vi "get display data.vi"(0 "display queues":T4, 1 "prune?":bool=TRUE, 5 "time range":dbl=-1.0, 9 "t0":dbl, 11 "error in (no error)":errorcluster, 12 "recent crossing":dbl) -> (4 "voltage graph":cluster{dbl[], dbl[]}, 6 "coil graph":cluster{dbl[], dbl[]}, 8 "pulse statistics":T1, 10 "extracted magnetism":T2[](array[typedef]), 15 "error out":errorcluster)   [LabVIEW 2017]
uses:
  typedefs/queue cluster.ctl
  typedefs/reading queue.ctl
  typedefs/reading.ctl
  typedefs/readingType.ctl
  typedefs/reading1.ctl
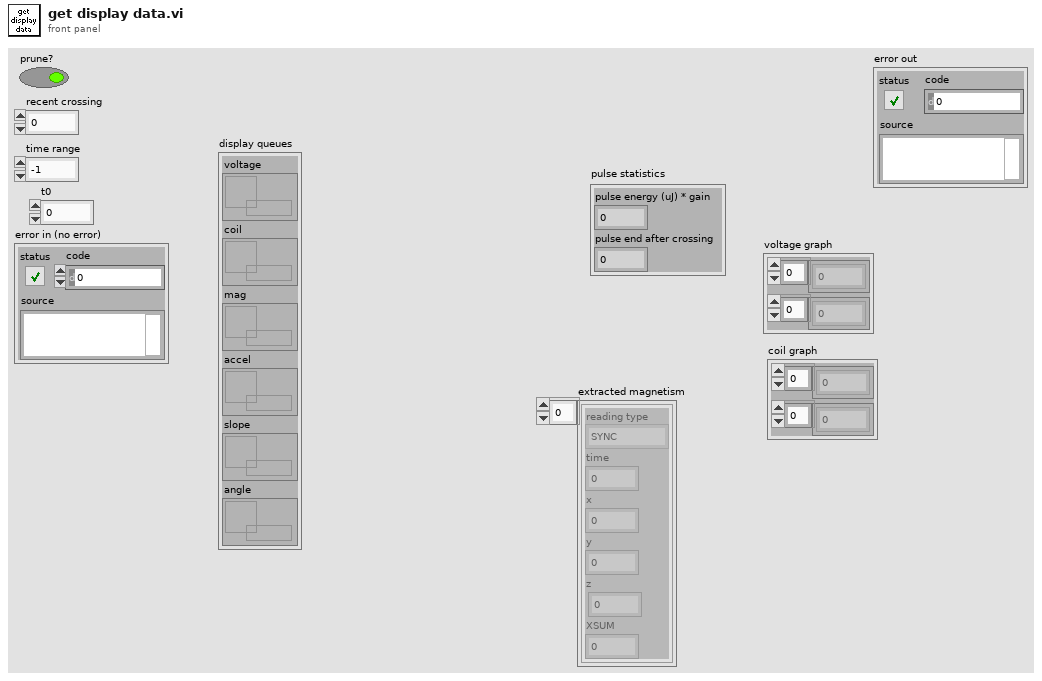
[diagram p1: front panel]
types:
  T1 = cluster{"pulse energy (uJ) * gain":sgl, "pulse end after crossing":dbl}
  T2 = typedef "reading.ctl" = cluster{"reading type":T3, "time":fxp<+,48,48>, "x":sgl, "y":sgl, "z":sgl, "XSUM":u8}
  T3 = typedef "readingType.ctl" = enum8{"SYNC", "DETVAL", "COILI", "MAGVEC", "ACCVEC"}
  T4 = typedef "queue cluster.ctl" = cluster{"voltage":T5, "coil":T5, "mag":T5, "accel":T5, "slope":refnum<queue>, "angle":refnum<queue>}
  T5 = typedef "reading queue.ctl" = refnum<queue>
  T6 = cluster{"tx":cluster{dbl[], sgl[]}, "ty":cluster{dbl[], sgl[]}, "tz":cluster{dbl[], sgl[]}, "xy":cluster{sgl[], sgl[]}}
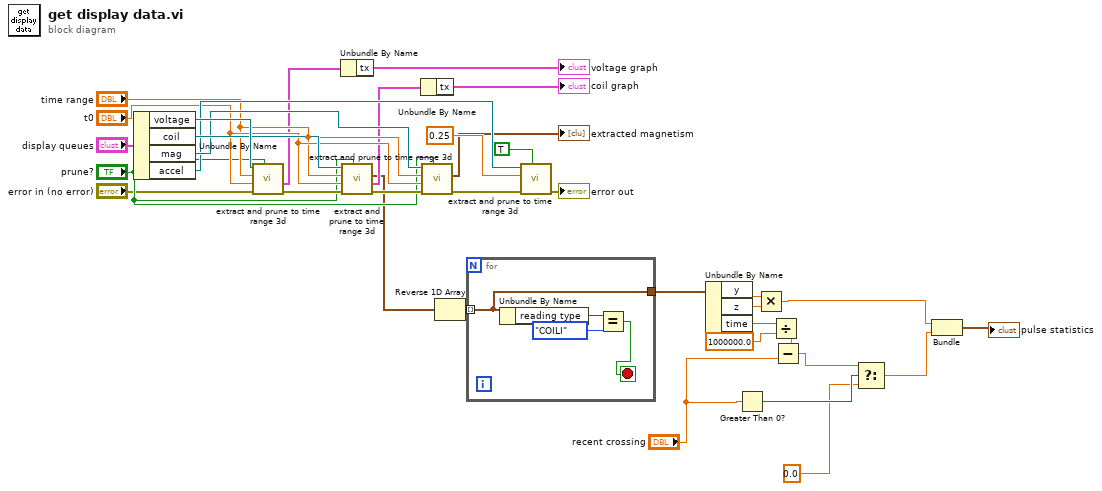
[diagram p0: block diagram]
diagram:
  n1 = Unbundle By Name("display queues") -> ("voltage"=w32:T5, "coil"=w31:T5, "mag"=w30:T5, "accel"=w29:T5)
  n2 = call "extract and prune to time range 3d.vi"("prune?"="prune?", "error in (no error)"="error in (no error)", "t0 (s)"="t0", "time range (s)"="time range", "queue in"=w32) -> ("error out"=w34:errorcluster, "graphs"=w19:T6)  [unwired: 3 in, 2 out]
  n3 = Unbundle By Name(w19) -> ("tx"=→"voltage graph":cluster{dbl[], sgl[]})
  n4 = call "extract and prune to time range 3d.vi"("prune?"="prune?", "error in (no error)"=w34, "t0 (s)"="t0", "time range (s)"="time range", "queue in"=w31) -> ("error out"=w28:errorcluster, "graphs"=w17:T6, "extracted data"=w15:T2[])  [unwired: 3 in, 1 out]
  n5 = Unbundle By Name(w17) -> ("tx"=→"coil graph":cluster{dbl[], sgl[]})
  n6 = call "extract and prune to time range 3d.vi"("prune?"="prune?", "error in (no error)"=w28, "t0 (s)"="t0", "time range (s)"="time range", "queue in"=w30) -> ("error out"=w27:errorcluster, "extracted data"=→"extracted magnetism":T2[])  [unwired: 3 in, 2 out]
  n7 = Reverse 1D Array(array=w15) -> (reversed array=w14:T2[])
  n8 = for {
    tunnel: w14 -> [w36] mode=indexing
    tunnel: [w36] -> w13
    stop <- w37 stop-if-true
    n9 = Unbundle By Name(w36) -> ("reading type"=w39:T3)
    n10 = Equal?(x=w39, y=readingType."COILI") -> (x = y?=w37:bool)
  }
  n11 = call "extract and prune to time range 3d.vi"("prune?"=TRUE, "error in (no error)"=w27, "time range (s)"=0.25 ("time range"), "queue in"=w29) -> ("error out"=→"error out":errorcluster)  [unwired: 4 in, 3 out]
  n12 = Unbundle By Name(w13) -> ("y"=w12:sgl, "z"=w11:sgl, "time"=w10:fxp<+,48,48>)
  n13 = Greater Than 0?(x="recent crossing") -> (x > 0?=w7:bool)
  n14 = Multiply(x=w12, y=w11) -> (x*y=w5:sgl)
  n15 = Divide(x=w10, y=1000000.0) -> (x/y=w2:dbl)
  n16 = Subtract(x=w2, y="recent crossing") -> (x-y=w8:dbl)
  n17 = Select(t=w8, s=w7, f=0.0) -> (s? t:f=w4:dbl)
  n18 = Bundle(w5, "f"=w4) -> (→"pulse statistics":cluster{sgl, "f":dbl})  [unwired: 1 in]
